vi "Image Processing Main Pipeline.vi"() -> ()   [LabVIEW 2009]
uses:
  <vilib>/vision/driver/NI_Vision_Acquisition_Software.lvlib
  <vilib>/vision/driver/IMAQdx.llb/IMAQdx Acquisition Mode.ctl
  <vilib>/userDefined/High Color/IMAQdx.ctl
panel:
  out "Sick array":i32[](array[numeric])
  out "x-y":u32
  in  "stop":bool
  out "Right Camera Input":T1(plugin-control)
  out "Left Camera Input":T1(plugin-control)
  out "Right Camera Output":T1(plugin-control)
  out "Left Camera Output":T1(plugin-control)
  in  "IMAQdx Session Right":T2="cam1" caption="Session In"
  in  "IMAQdx Session Left":T2="cam0" caption="Session In"
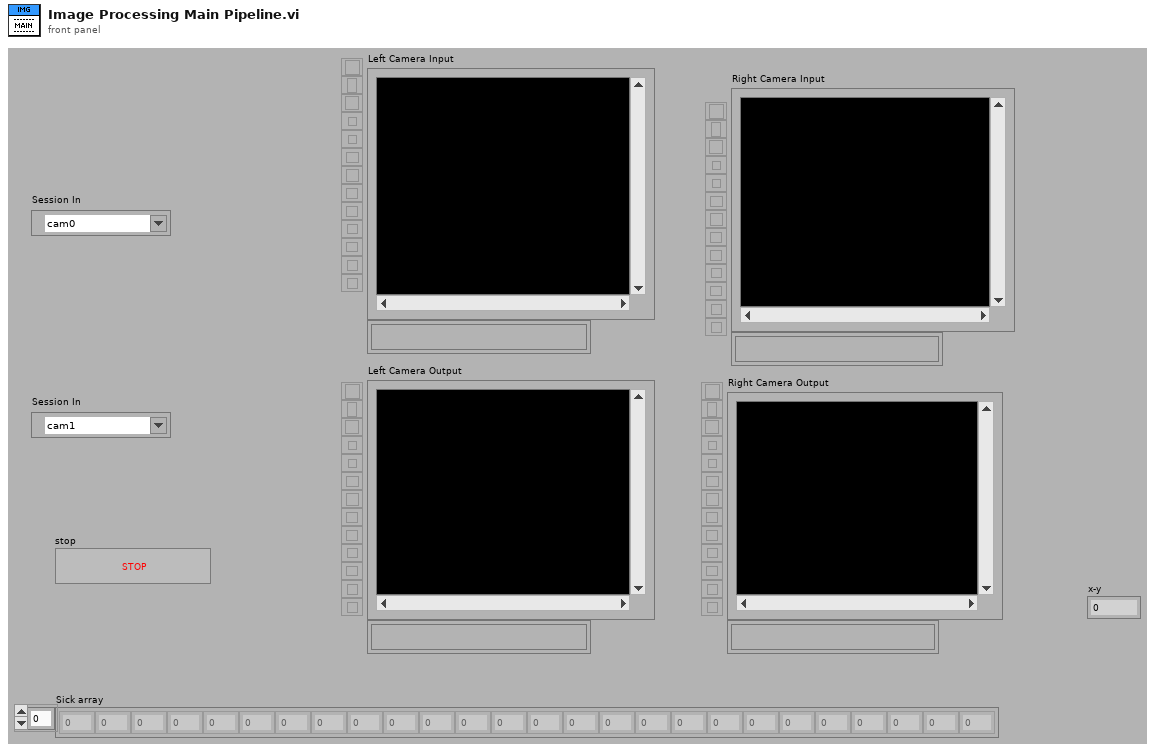
[diagram p1: front panel]
types:
  T1 = typedef "IMAQ Image.ctl" = refnum<image>
  T2 = typedef "IMAQdx.ctl" = refnum<k21>
  T3 = typedef "NI_Vision_Acquisition_Software.lvlib/IMAQdx Acquisition Mode.ctl" = enum32{"One Shot", "Continuous"}
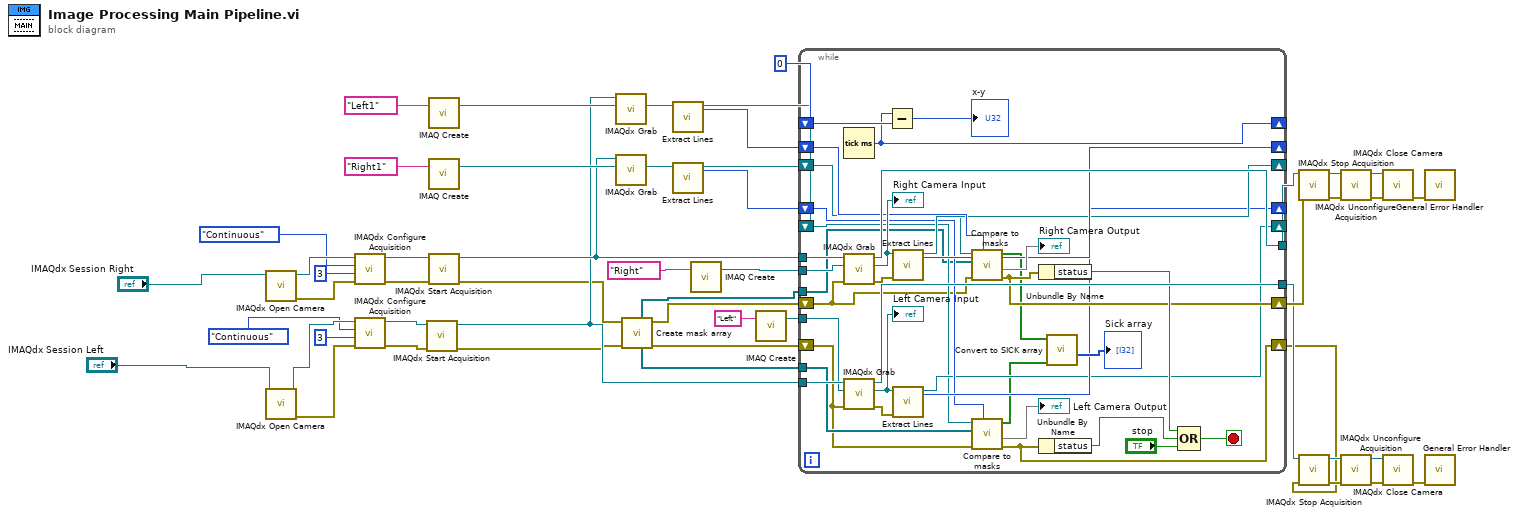
[diagram p0: block diagram]
diagram:
  n1 = call <vilib>:"IMAQdx Open Camera.vi"("Session In"="IMAQdx Session Right") -> ("error out"=w40:errorcluster, "Session Out"=w41:T2)  [unwired: 2 in, 7 out]
  n2 = call <vilib>:"IMAQdx Open Camera.vi"("Session In"="IMAQdx Session Left") -> ("error out"=w46:errorcluster, "Session Out"=w45:T2)  [unwired: 2 in, 7 out]
  n3 = call <vilib>:"IMAQdx Configure Acquisition.vi"("error in"=w40, "Number of Buffers"=u32 3, "Continuous?"=IMAQdx_Acquisition_Mode."Continuous", "Session In"=w41) -> ("error out"=w39:errorcluster, "Session Out"=w42:T2)  [unwired: 1 in, 5 out]
  n4 = call <vilib>:"IMAQdx Configure Acquisition.vi"("error in"=w46, "Number of Buffers"=u32 3, "Continuous?"=IMAQdx_Acquisition_Mode."Continuous", "Session In"=w45) -> ("error out"=w47:errorcluster, "Session Out"=w44:T2)  [unwired: 1 in, 5 out]
  n5 = call <vilib>:"IMAQdx Start Acquisition.vi"("error in"=w47, "Session In"=w44) -> ("error out"=w5:errorcluster, "Session Out"=w13:T2)  [unwired: 8 out]
  n6 = call "IMAQ Create"("Image Name"="Left1") -> ("New Image"=w15:T1)  [unwired: 4 in, 1 out]
  n7 = call "IMAQ Create"("Image Name"="Right1") -> ("New Image"=w16:T1)  [unwired: 4 in, 1 out]
  n8 = call <vilib>:"IMAQdx Start Acquisition.vi"("error in"=w39, "Session In"=w42) -> ("error out"=w6:errorcluster, "Session Out"=w14:T2)  [unwired: 8 out]
  n9 = call <vilib>:"IMAQdx Grab.vi"("Image In"=w15, "Session In"=w13) -> ("Image Out"=w8:T1)  [unwired: 6 in, 3 out]
  n10 = call <vilib>:"IMAQdx Grab.vi"("Image In"=w16, "Session In"=w14) -> ("Image Out"=w11:T1)  [unwired: 6 in, 3 out]
  n11 = call "Create mask array.vi"("Left error in"=w5, "Right Error in"=w6) -> ("Left error out"=w3:errorcluster, "Right error out"=w4:errorcluster, "Left Cam Masks"=w1:T1[], "Right Cam Masks"=w2:T1[])  [unwired: 6 in]
  n12 = call "Extract Lines.vi"("Image Src"=w8) -> ("Image Out"=w9:T1, "Extraction mode"=w7:i32)  [unwired: 7 in, 2 out]
  n13 = call "Extract Lines.vi"("Image Src"=w11) -> ("Image Out"=w12:T1, "Extraction mode"=w10:i32)  [unwired: 7 in, 2 out]
  n14 = call "IMAQ Create"("Image Name"="Right") -> ("New Image"=w50:T1)  [unwired: 4 in, 1 out]
  n15 = call "IMAQ Create"("Image Name"="Left") -> ("New Image"=w49:T1)  [unwired: 4 in, 1 out]
  n16 = while {
    tunnel: w13 -> [w87]
    tunnel: w49 -> [w86]
    tunnel: w14 -> [w85]
    tunnel: w50 -> [w84]
    tunnel: [w83] -> w25
    tunnel: [w82] -> w32
    shift-right: [w76] -> _
    shift-left: u32 0 -> [w77]
    shift-right: [w65] -> _
    shift-left: w7 -> [w64]
    shift-right: [w63] -> _
    shift-left: w9 -> [w62]
    shift-right: [w61] -> _
    shift-left: w10 -> [w60]
    shift-right: [w59] -> _
    shift-left: w12 -> [w58]
    tunnel: w2 -> [w57]
    tunnel: w1 -> [w56]
    shift-right: [w69] -> w31
    shift-left: w4 -> [w54]
    shift-right: [w70] -> w24
    shift-left: w3 -> [w55]
    stop <- w78 stop-if-true
    n17 = Tick Count (ms)() -> (millisecond timer value=w76:u32)
    n18 = call <vilib>:"IMAQdx Grab.vi"("error in"=w54, "Image In"=w84, "Session In"=w85) -> ("error out"=w73:errorcluster, "Image Out"=w74:T1, "Session Out"=w82:T2)  [unwired: 5 in, 1 out]
    "Right Camera Input" <- w74
    n19 = call <vilib>:"IMAQdx Grab.vi"("error in"=w55, "Image In"=w86, "Session In"=w87) -> ("error out"=w71:errorcluster, "Image Out"=w72:T1, "Session Out"=w83:T2)  [unwired: 5 in, 1 out]
    "Left Camera Input" <- w72
    n20 = Subtract(x=w76, y=w77) -> (x-y=→"x-y":u32)
    n21 = call "Extract Lines.vi"("error in (no error)"=w73, "Image Src"=w74) -> ("Image Out"=w63:T1, "Extraction mode"=w65:i32)  [unwired: 6 in, 2 out]
    n22 = call "Extract Lines.vi"("error in (no error)"=w71, "Image Src"=w72) -> ("Image Out"=w59:T1, "Extraction mode"=w61:i32)  [unwired: 6 in, 2 out]
    n23 = call "Compare to masks.vi"("Number of Particles1"=w64, "error in (no error)"=w54, "Mask array"=w57, "Image Src"=w62) -> ("Final error out"=w69:errorcluster, 1:→"Right Camera Output", "Marked Regions"=w53:bool[])  [unwired: 5 in]
    n24 = call "Compare to masks.vi"("Number of Particles1"=w60, "error in (no error)"=w55, "Mask array"=w56, "Image Src"=w58) -> ("Final error out"=w70:errorcluster, 1:→"Left Camera Output", "Marked Regions"=w52:bool[])  [unwired: 5 in]
    n25 = Unbundle By Name(w69) -> ("status"=w81:bool)
    n26 = Unbundle By Name(w70) -> ("status"=w80:bool)
    n27 = call "Convert to SICK array.vi"("Left Regions"=w52, "Right Regions"=w53) -> ("Sick array"=→"Sick array":u16[])  [unwired: 9 in]
    n28 = Compound Arithmetic op=OR(w81, w80, "stop") -> (w78:bool)
  }
  n29 = call <vilib>:"IMAQdx Stop Acquisition.vi"("error in"=w31, "Session In"=w32) -> ("error out"=w35:errorcluster, "Session Out"=w34:T2)  [unwired: 8 out]
  n30 = call <vilib>:"IMAQdx Stop Acquisition.vi"("error in"=w24, "Session In"=w25) -> ("error out"=w28:errorcluster, "Session Out"=w29:T2)  [unwired: 8 out]
  n31 = call <vilib>:"IMAQdx Unconfigure Acquisition.vi"("error in"=w35, "Session In"=w34) -> ("error out"=w36:errorcluster, "Session Out"=w37:T2)  [unwired: 8 out]
  n32 = call <vilib>:"IMAQdx Unconfigure Acquisition.vi"("error in"=w28, "Session In"=w29) -> ("error out"=w27:errorcluster, "Session Out"=w26:T2)  [unwired: 8 out]
  n33 = call <vilib>:"IMAQdx Close Camera.vi"("error in"=w36, "Session In"=w37) -> ("error out"=w33:errorcluster)  [unwired: 9 out]
  n34 = call <vilib>:"IMAQdx Close Camera.vi"("error in"=w27, "Session In"=w26) -> ("error out"=w30:errorcluster)  [unwired: 9 out]
  n35 = call <vilib>:"General Error Handler.vi"("error in (no error)"=w33) -> ()  [unwired: 1 in, 14 out]
  n36 = call <vilib>:"General Error Handler.vi"("error in (no error)"=w30) -> ()  [unwired: 1 in, 14 out]
